vi "Indicate Valves.vi"(8 "error in (no error)":errorcluster, 10 "Numeric":u16, 11 "Storage in":refnum<class "Storage.lvclass">) -> (0 "error out":errorcluster, 3 "Storage out":refnum<class "Storage.lvclass">)   [LabVIEW 2015, in "AMS UI.lvlib" / "Storage.lvclass"]
uses:
  Storage.lvclass
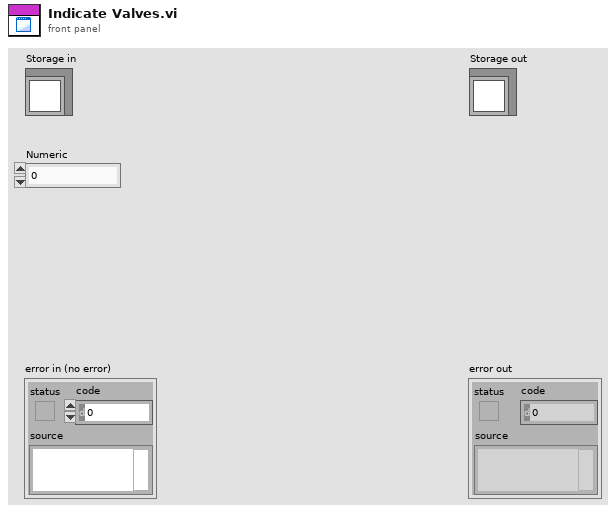
[diagram p1: front panel]
types:
  T1 = typedef "FP Control Refs Cluster.ctl" = cluster{"Liquid N Valve References":T2, "Main Line Valve Refs":T3, "Transfer Line Container":refnum<vi>, "Storage Containers":refnum<vi>[], "Sample Refs":T4, "Syringe Ctrl Refs ":T5, "Baratrons Chart":refnum<vi>, "Capillary Container":refnum<vi>, "Preparation Container":refnum<vi>, "Monkey Mode":refnum<vi>}
  T2 = typedef "Liquid N Valve Ref Cluster.ctl" = cluster{"Cold Bath H2O HV 100":refnum<vi>, "Cold Bath Cleaning HV 101":refnum<vi>, "Cold Bath Storage 1 HV 102":refnum<vi>, "Cold Bath Storage 2 HV 103":refnum<vi>, "Cold Bath Storage 3 HV 104":refnum<vi>, "Cold Bath Storage 4 HV 105":refnum<vi>, "Cold Bath Syringe HV 106":refnum<vi>, "Liquid N Master Valve HV 107":refnum<vi>}
  T3 = typedef "Main Line Valve Ref Cluster.ctl" = cluster{"Turbo Valve DV313":refnum<vi>, "Prep Line Valve 0 DV300":refnum<vi>, "Storage Valves":refnum<vi>[]}
  T4 = typedef "Sample Valve Refs.ctl" = cluster{"Valves":cluster{"Sample 5 DV318":refnum<vi>, "Sample 4 DV317":refnum<vi>, "Sample 3 DV316":refnum<vi>, "Sample 2 DV315":refnum<vi>, "Sample 1 DV314":refnum<vi>}, "Lines":cluster{"Sample 1":refnum<vi>, "Sample 2":refnum<vi>, "Sample 3":refnum<vi>, "Sample 4":refnum<vi>, "Sample 5":refnum<vi>}}
  T5 = typedef "Syringe Ctrl Refs.ctl" = cluster{"Syringe Home":refnum<vi>, "Syringe Freeze":refnum<vi>, "Syringe TC":refnum<vi>, "Syringe Container":refnum<vi>}
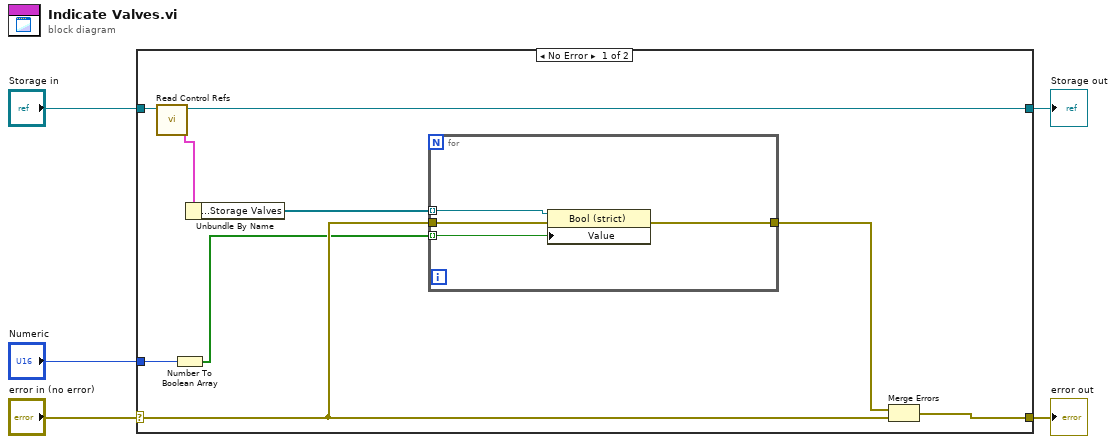
[diagram p0: block diagram]
diagram:
  n1 = case shown="No Error" "error in (no error)" {
    selector: "error in (no error)" -> [w9 w20]
    tunnel: [w10 w20] -> w4
    tunnel: [w11 w19] -> w2
    tunnel: "Storage in" -> [w12 w19]
    tunnel: "Numeric" -> [w14 _]
    frame No Error {
      n2 = call-dynamic "Read Control Refs.vi"("AMS Gas Actor in"=w12) -> ("Control Refs"=w13:T1, "AMS Gas Actor out"=w11:refnum<class "Storage.lvclass">)  [unwired: 9 in]
      n3 = Number To Boolean Array(number=w14) -> (Boolean array=w7:bool[])
      n4 = Unbundle By Name(w13) -> ("Main Line Valve Refs.Storage Valves"=w6:refnum<vi>[])
      n5 = for {
        tunnel: w7 -> [w16] mode=indexing
        tunnel: w6 -> [w18] mode=indexing
        tunnel: w9 -> [w15]
        tunnel: [w17] -> w8
        n6 = property class="Bool (strict)"(reference=w18, error in=w15, "Value"=w16) -> (error out=w17:errorcluster)  [unwired: 1 out]
      }
      n7 = Merge Errors(w8, w9) -> (w10:errorcluster)
    }
    frame Error {
    }
  }
  "error out" <- w4
  "Storage out" <- w2
